vi "best linear fit.vi"() -> ()   [LabVIEW 2020]
uses:
  <vilib>/Analysis/NI_AALPro.lvlib
panel:
  out "intercept":dbl
  out "slope":dbl
  out "Wielomian najlepszego dopasowania":dbl[][](graph)
  in  "k":dbl
  in  "N":i32
  in  "Faza":dbl
  in  "Amplituda":dbl
  out "Prosta najlepszego dopasowania":dbl[][](graph)
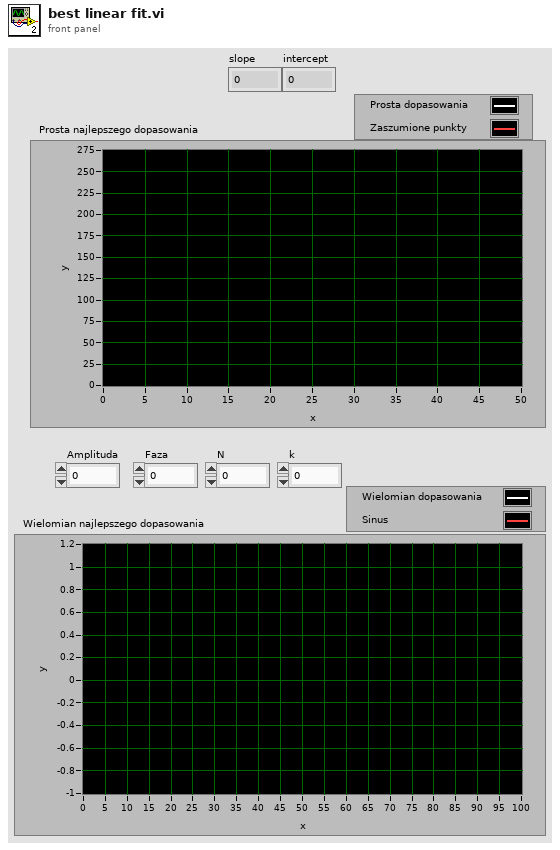
[diagram p1: front panel]
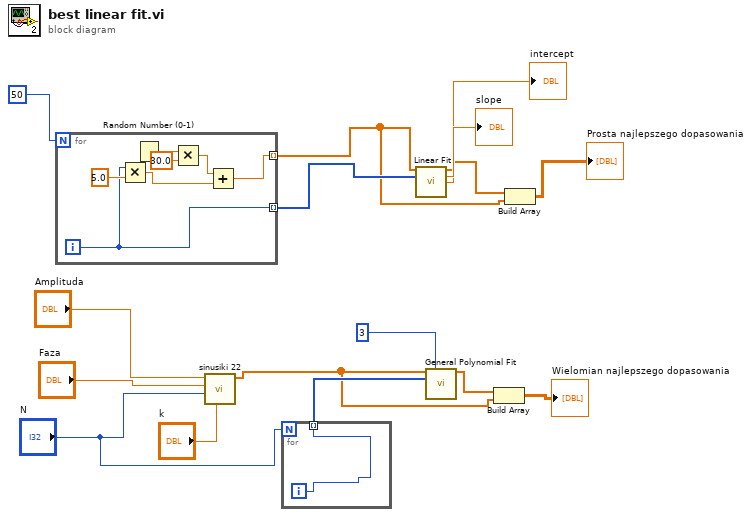
[diagram p0: block diagram]
diagram:
  n1 = for {
    N: 50 -> [_]
    tunnel: [w20] -> w4 mode=indexing
    tunnel: [w22] -> w8 mode=indexing
    i -> [w22]
    n2 = Multiply(x=w22, y=5.0) -> (x*y=w21:dbl)
    n3 = Random Number (0-1)() -> (number: 0 to 1=w19:dbl)
    n4 = Multiply(x=w19, y=30.0) -> (x*y=w17:dbl)
    n5 = Add(x=w17, y=w21) -> (x+y=w20:dbl)
  }
  n6 = call "sinusiki 22.vi"("k"="k", "N"="N", "Faza"="Faza", "Amplituda"="Amplituda") -> ("Array"=w1:dbl[])  [unwired: 7 in]
  n7 = for {
    N: "N" -> [_]
    tunnel: [w24] -> w11 mode=indexing
    i -> [w24]
  }
  n8 = call <vilib>:"Linear Fit.vi"("Y"=w4, "X"=w8) -> ("Best Linear Fit"=w6:dbl[], "slope"=→"slope":dbl, "intercept"=→"intercept":dbl)  [unwired: 9 in, 2 out]
  n9 = call <vilib>:"General Polynomial Fit.vi"("Y"=w1, "polynomial order"=3, "X"=w11) -> ("Best Polynomial Fit"=w3:dbl[])  [unwired: 9 in, 3 out]
  n10 = Build Array(w3, w1) -> (→"Wielomian najlepszego dopasowania":dbl[][])
  n11 = Build Array(w6, w4) -> (→"Prosta najlepszego dopasowania":dbl[][])
